vi "create polynomial curve form coeffs (SubVI).vi"(9 "Polynomial Coefficients":dbl[](array[numeric]), 10 "input data":dbl[](array[numeric]), 11 "# of data points":u32=10000) -> (3 "Cluster":cluster{dbl[], dbl[]})   [LabVIEW 2024]
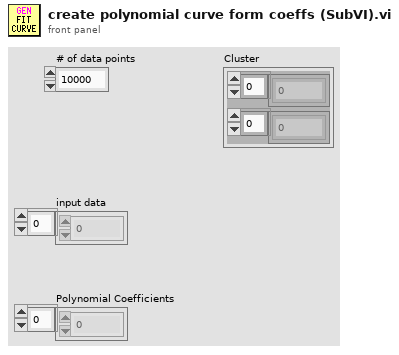
[diagram p1: front panel]
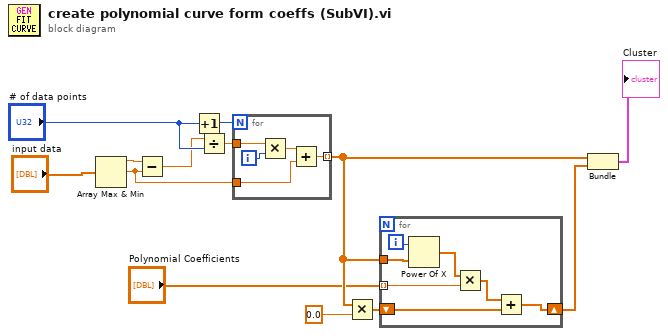
[diagram p0: block diagram]
diagram:
  n1 = Array Max & Min(array="input data") -> (max value=w3:dbl, min value=w5:dbl)  [unwired: 2 out]
  n2 = Subtract(x=w3, y=w5) -> (x-y=w4:dbl)
  n3 = Increment(x="# of data points") -> (x+1=w7:u32)
  n4 = Divide(x=w4, y="# of data points") -> (x/y=w6:dbl)
  n5 = for {
    N: w7 -> [_]
    tunnel: w5 -> [w15]
    tunnel: w6 -> [w18]
    tunnel: [w14] -> w12 mode=indexing
    i -> [w17]
    n6 = Multiply(x=w18, y=w17) -> (x*y=w16:dbl)
    n7 = Add(x=w16, y=w15) -> (x+y=w14:dbl)
  }
  n8 = Multiply(x=w12, y=0.0) -> (x*y=w13:dbl[])
  n9 = for {
    tunnel: "Polynomial Coefficients" -> [w22] mode=indexing
    tunnel: w12 -> [w25]
    shift-right: [w19] -> w9
    shift-left: w13 -> [w20]
    i -> [w24]
    n10 = Power Of X(1:w25, 2:w24) -> (0:w23:dbl[])
    n11 = Multiply(x=w23, y=w22) -> (x*y=w21:dbl[])
    n12 = Add(x=w21, y=w20) -> (x+y=w19:dbl[])
  }
  n13 = Bundle(w12, w9) -> (→"Cluster":cluster{dbl[], dbl[]})  [unwired: 1 in]
